vi "callback on WriteTree.vi"(8 "error in":errorcluster, 11 "node":refnum<data-value>) -> (0 "error out":errorcluster)   [LabVIEW 2013, in "NISE_CEF_serializable node.lvclass"]
uses:
  NISE_CEF_serializable node.lvclass
  Node/NISE_CEF_Node.lvclass
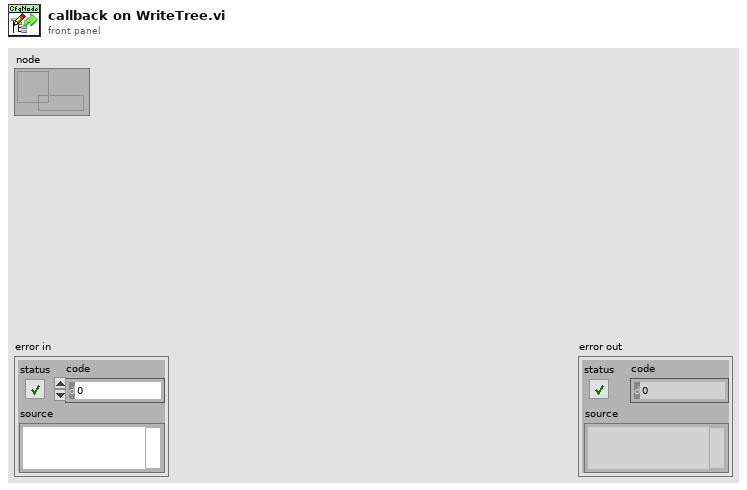
[diagram p1: front panel]
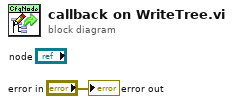
[diagram p0: block diagram]
diagram:
  "error out" <- "error in"
